vi "Meter Detection Main Page.vi"(8 "error in (no error)":errorcluster, 11 "Node Ptr":T2 format="%.0x") -> (0 "error out":errorcluster)   [LabVIEW 2011, in "Meter Detection Custom Device.lvlib"]
uses:
  Meter Detection Custom Device.lvlib
  <vilib>/NI Veristand/Custom Device API/Custom Device Item Ref.ctl
  <vilib>/NI Veristand/Custom Device API/Custom Device API.lvlib
  <vilib>/vision/driver/NI_Vision_Acquisition_Software.lvlib
panel:
  in  "Needle Configuration":bool
  in  "Reset Max":bool
  in  "Max Meter Value":dbl
  in  "Set Max Meter ROI":bool
  out "Instructions for Use":string
  in  "Reset Min":bool
  in  "Min Meter Value":dbl
  in  "Camera Interface":string
  in  "Set Min Meter ROI":bool
  in  "Capture Image":bool
  out "Image":T1(plugin-control)
  in  "Header":cluster{"Section Name":string}={"Section Name"="Custom Device Item Settings"}
  in  "Name":string
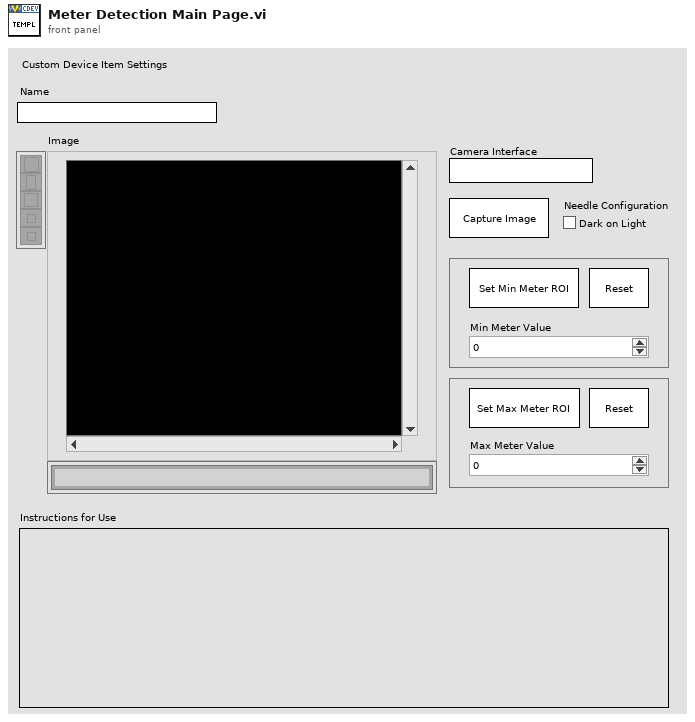
[diagram p1: front panel]
types:
  T1 = typedef "IMAQ Image.ctl" = refnum<image>
  T2 = typedef "Custom Device API.lvlib/Custom Device Item Ref.ctl" = u64
  T3 = typedef "Custom Device API.lvlib/Custom Device Item Info.ctl" = cluster{"Name":string, "Is Channel":bool, "GUID":string}
  T4 = typedef "IMAQdx.ctl" = refnum<k21>
  T5 = cluster{"Global Rectangle":i32[], "Contours":cluster{"Contour Type":u32, "ROI Type":u32, "Points":i32[]}[]}
  T6 = typedef "Custom Device API.lvlib/Custom Device Commands.ctl" = enum16{"Default", "Item renamed", "Shutdown", "Dynamic button pressed"}
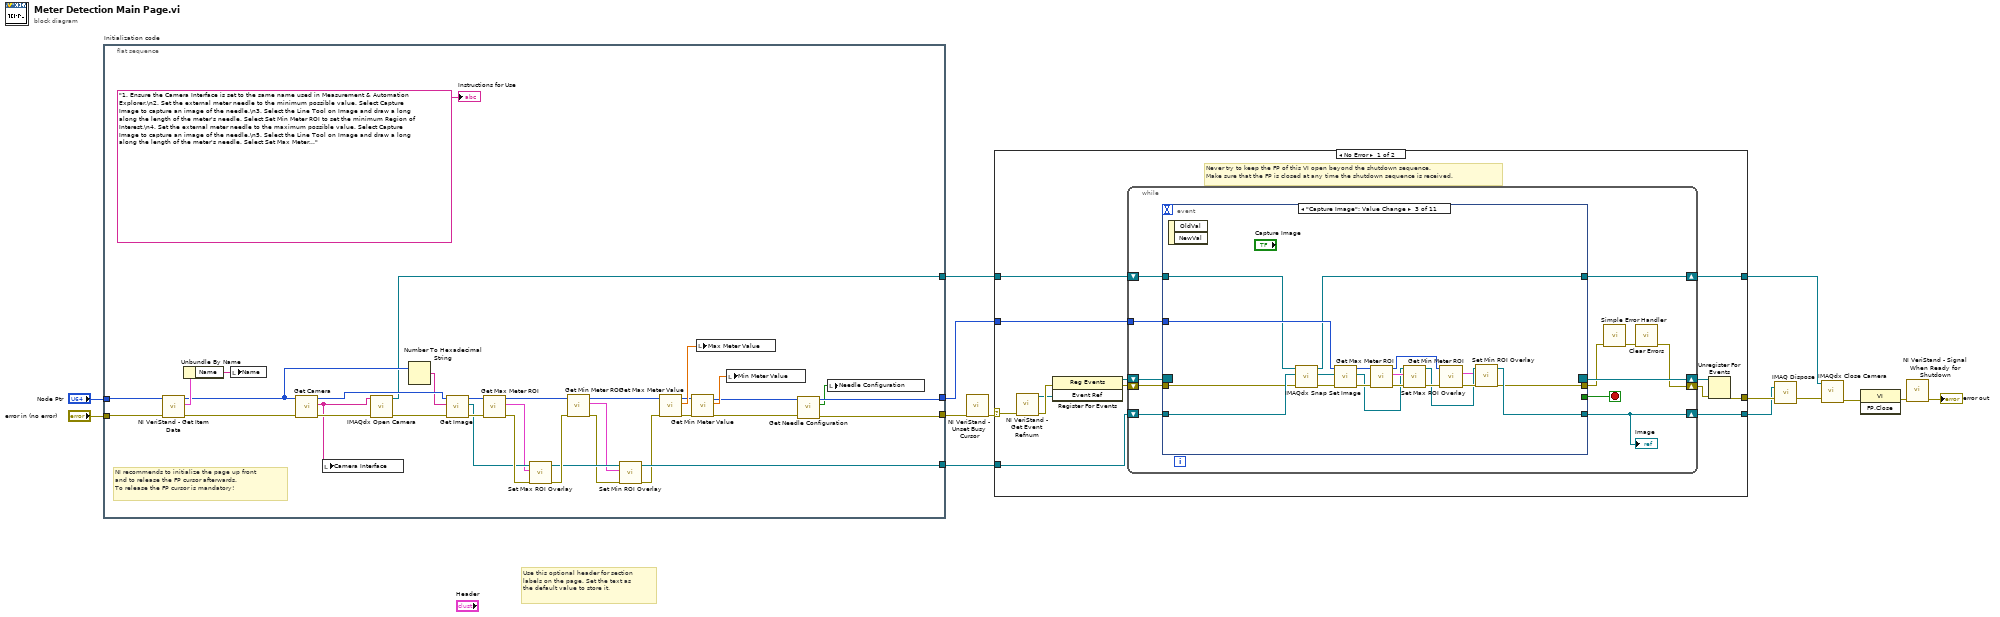
[diagram p0: block diagram]
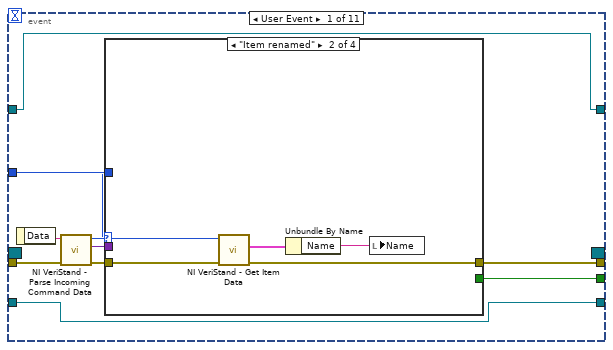
[diagram p2: hidden frame]
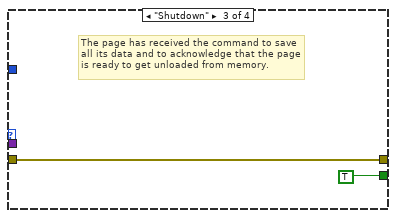
[diagram p4: hidden frame]
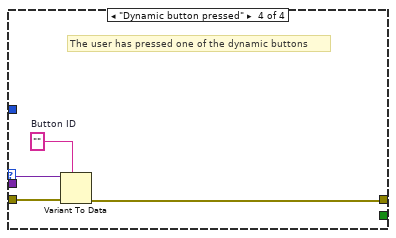
[diagram p5: hidden frame]
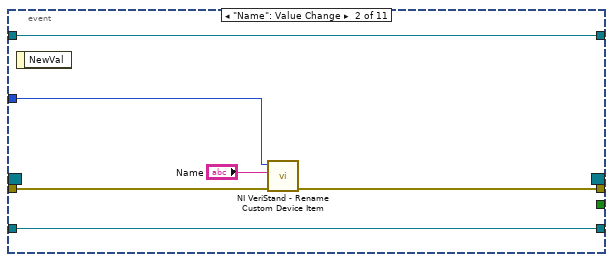
[diagram p6: hidden frame]
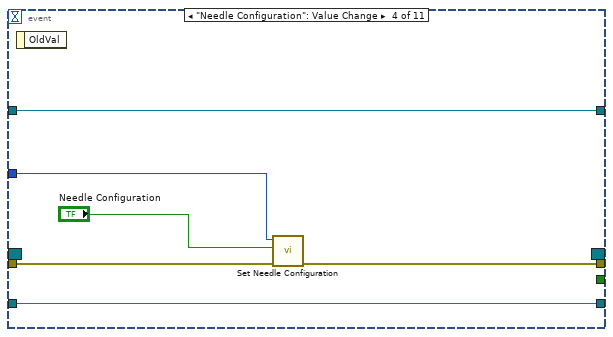
[diagram p7: hidden frame]
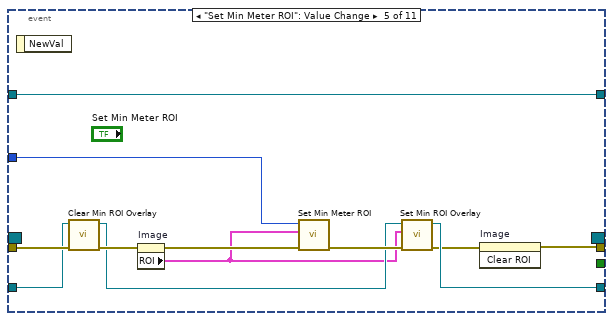
[diagram p8: hidden frame]
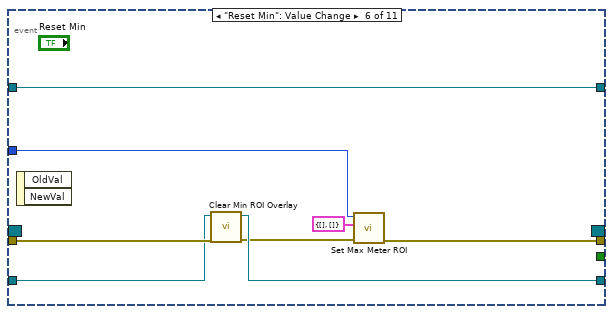
[diagram p9: hidden frame]
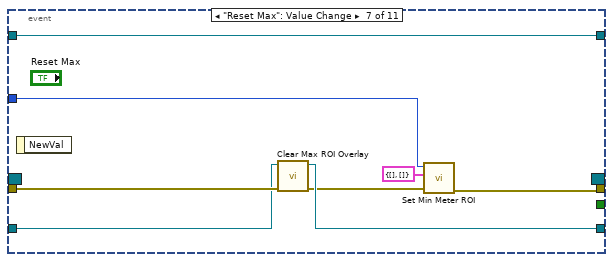
[diagram p10: hidden frame]
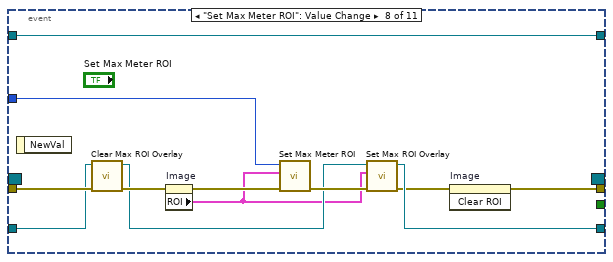
[diagram p11: hidden frame]
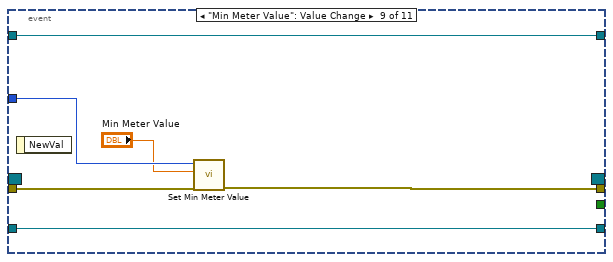
[diagram p12: hidden frame]
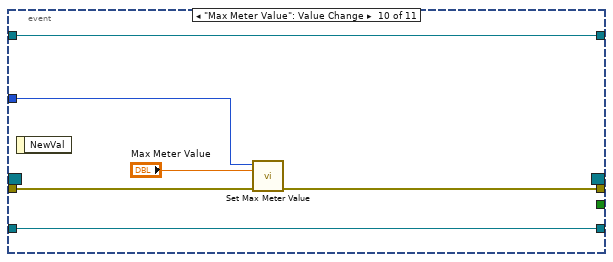
[diagram p13: hidden frame]
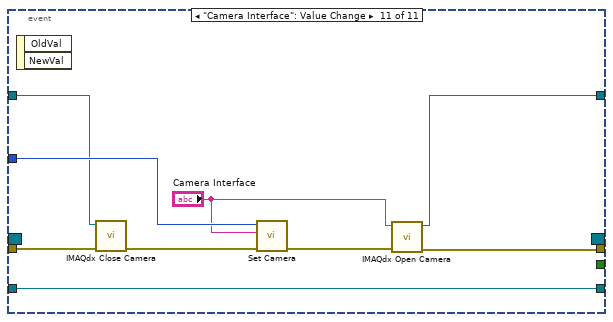
[diagram p14: hidden frame]
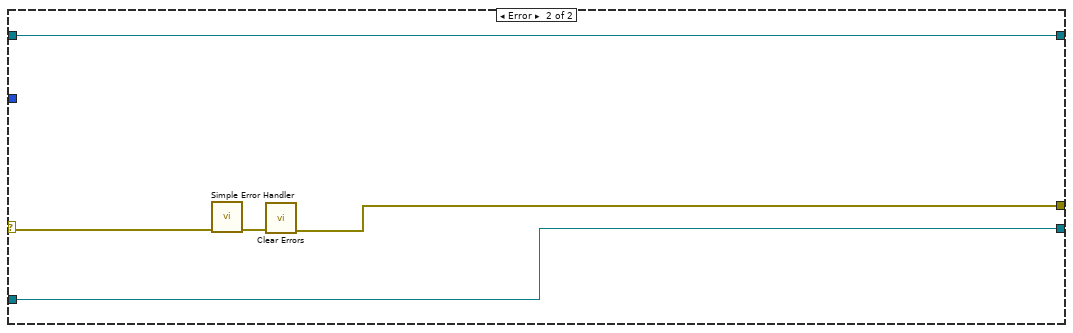
[diagram p15: hidden frame]
diagram:
  # "Use this optional header for section labels on the page. Set the text as the default value to store it."
  n1 = flat-sequence "Initialization code" {
    tunnel: "error in (no error)" -> [w46]
    tunnel: "Node Ptr" -> [w47]
    tunnel: [w16] -> w11
    tunnel: [w17] -> w8
    tunnel: [w27] -> w5
    tunnel: [w21] -> w4
    frame #0 {
      # "NI recommends to initialize the page up front\nand to release the FP cursor afterwards.\nTo release the FP cursor is mandatory!"
      n2 = call <vilib>:"NI VeriStand - Get Item Data.vi"("error in (no error)"=w46, "Item Ref in"=w47) -> ("error out"=w45:errorcluster, "Item Info"=w49:T3, "Item Ref out"=w41:T2)  [unwired: 7 out]
      n3 = Unbundle By Name(w49) -> ("Name"=w48:string)
      n4 = local write "Name"(w48) -> ()
      n5 = call "Get Camera.vi"("error in (no error)"=w45, "Item Ref out in"=w41) -> ("error out"=w24:errorcluster, "Camera"=w22:string, "Item Ref out out"=w44:T2)  [unwired: 7 in]
      n6 = local write "Camera Interface"(w22) -> ()
      n7 = call <vilib>:"IMAQdx Open Camera.vi"("error in"=w24, "Session In"=w22) -> ("error out"=w23:errorcluster, "Session Out"=w21:T4)  [unwired: 8 in]
      n8 = Number To Hexadecimal String(2:w41) -> (0:w35:string)  [unwired: 1 in]
      n9 = call "Get Image.vi"("error in (no error)"=w23, "Image Name"=w35, "Item Ref out out"=w44) -> ("error out"=w34:errorcluster, "Image out"=w31:T1, "Item Ref out"=w43:T2)  [unwired: 5 in, 1 out]
      n10 = call "Get Max Meter ROI.vi"("error in (no error)"=w34, "Item Ref in"=w43) -> ("error out"=w33:errorcluster, "Max Gauge ROI"=w30:T5, "Item Ref out"=w40:T2)  [unwired: 6 in, 1 out]
      n11 = call "Set Max ROI Overlay.vi"("error in (no error)"=w33, "Max Gauge ROI"=w30, "Image in"=w31) -> ("error out"=w32:errorcluster, "Image out"=w29:T1)  [unwired: 7 in]
      n12 = call "Get Min Meter ROI.vi"("error in (no error)"=w32, "Item Ref in"=w40) -> ("error out"=w28:errorcluster, "Max Gauge ROI"=w25:T5, "Item Ref out"=w39:T2)  [unwired: 6 in, 1 out]
      n13 = call "Set Min ROI Overlay.vi"("error in (no error)"=w28, "Min Gauge ROI"=w25, "Image in"=w29) -> ("error out"=w26:errorcluster, "Image out"=w27:T1)  [unwired: 7 in]
      n14 = call "Get Max Meter Value.vi"("error in (no error)"=w26, "Item Ref in"=w39) -> ("error out"=w38:errorcluster, "Max Gauge Value"=w42:dbl, "Item Ref out"=w37:T2)  [unwired: 7 in]
      n15 = call "Get Min Meter Value.vi"("error in (no error)"=w38, "Item Ref in"=w37) -> ("error out"=w19:errorcluster, "Min Gauge Value"=w36:dbl, "Item Ref out"=w18:T2)  [unwired: 7 in]
      n16 = local write "Max Meter Value"(w42) -> ()
      n17 = local write "Min Meter Value"(w36) -> ()
      n18 = call "Get Needle Configuration.vi"("error in (no error)"=w19, "Item Ref in"=w18) -> ("error out"=w16:errorcluster, "Needle Configuration out"=w15:bool, "Item Ref out"=w17:T2)  [unwired: 7 in]
      n19 = local write "Needle Configuration"(w15) -> ()
      "Instructions for Use" <- "1. Ensure the Camera Interface is set to the same name used in Measurement & Automation Explorer.\n2. Set the external meter needle to the minimum possible value. Select Capture Image to capture an image of the needle.\n3. Select the Line Tool on Image and draw a long along the length of the meter's needle. Select Set Min Meter ROI to set the minimum Region of Interest.\n4. Set the external meter needle to the maximum possible value. Select Capture Image to capture an image of the needle.\n5. Select the Line Tool on Image and draw a long along the length of the meter's needle. Select Set Max Meter ROI to set the maximum Region of Interest.\n6. Ensure the Min Meter Value and Max Meter Value correspond to the minimum and maximum possible meter values respectively and set the Needle Configuration appropriately.\n7. Save the system definition file. " ("Directions")
    }
  }
  n20 = call <vilib>:"NI VeriStand - Unset Busy Cursor.vi"("error in (no error)"=w11) -> ("error out"=w10:errorcluster)  [unwired: 10 out]
  n21 = case shown="No Error" w10 {
    selector: w10 -> [w54 w193]
    tunnel: [w59 w191] -> w7
    tunnel: w8 -> [w55 _]
    tunnel: [w53 w190] -> w6
    tunnel: w5 -> [w52 w190]
    tunnel: w4 -> [w51 w189]
    tunnel: [w50 w189] -> w1
    frame No Error {
      # "Never try to keep the FP of this VI open beyond the shutdown sequence.\nMake sure that the FP is closed at any time the shutdown sequence is received."
      n22 = call <vilib>:"NI VeriStand - Get Event Refnum.vi"("error in (no error)"=w54) -> ("error out"=w62:errorcluster, "Event Ref"=w58:refnum<user-event>)  [unwired: 9 out]
      n23 = register-events(error in=w62, w58) -> (reference out=w56:refnum<event-registration>, error out=w57:errorcluster)  [unwired: 1 in]
      n24 = while {
        tunnel: w55 -> [w70]
        shift-right: [w67] -> w60
        shift-left: w57 -> [w73]
        shift-right: [w74] -> w61
        shift-left: w56 -> [w72]
        shift-right: [w65] -> w53
        shift-left: w52 -> [w66]
        shift-right: [w63] -> w50
        shift-left: w51 -> [w64]
        stop <- w71 stop-if-true
        n25 = event shown="[2] \"Capture Image\": Value Change" {
          selector: w72 -> [_ _ _ _ _ _ _ _ _ _ _]
          dyn-events: [_ _ _ _ _ _ _ _ _ _ _] -> w74
          timeout: _ -> [_ _ _ _ _ _ _ _ _ _ _]
          tunnel: w73 -> [w84 w102 w105 w124 w137 w147 w155 w165 w170 w178 w186]
          tunnel: [w80 _ _ _ _ _ _ _ _ _ _] -> w71
          tunnel: [w79 w101 w104 w123 w129 w143 w151 w157 w171 w177 w180] -> w69
          tunnel: w70 -> [w78 w100 w119 w125 w138 w142 w150 w166 w172 w175 w188]
          tunnel: w66 -> [w76 w98 w121 w122 w135 w146 w154 w163 w173 w179 w187]
          tunnel: [w76 w98 w107 w122 w132 w145 w153 w160 w173 w179 w187] -> w65
          tunnel: w64 -> [w75 w97 w106 w127 w128 w140 w148 w156 w168 w174 w184]
          tunnel: [w75 w97 w103 w127 w128 w140 w148 w156 w168 w174 w181] -> w63
          event User Event {
            n26 = event-data() -> ("Data"=w83:string)  [unwired: 1 out]
            n27 = call <vilib>:"NI VeriStand - Parse Incoming Command Data.vi"("error in (no error)"=w84, "Incoming data"=w83) -> ("error out"=w82:errorcluster, "Outgoing data"=w77:variant, "Action"=w81:T6)  [unwired: 7 out]
            n28 = case shown="\"Item renamed\"" w81 {
              tunnel: w82 -> [w85 w90 w91 w96]
              tunnel: [_ _ TRUE _] -> w80
              tunnel: [w85 w87 w91 w93] -> w79
              tunnel: w78 -> [_ w89 _ _]
              tunnel: w77 -> [_ _ _ w95]
              frame "Default", Default {
              }
              frame "Item renamed" {
                n29 = call <vilib>:"NI VeriStand - Get Item Data.vi"("error in (no error)"=w90, "Item Ref in"=w89) -> ("error out"=w87:errorcluster, "Item Info"=w88:T3)  [unwired: 8 out]
                n30 = Unbundle By Name(w88) -> ("Name"=w86:string)
                n31 = local write "Name"(w86) -> ()
              }
              frame "Shutdown" {
                # "The page has received the command to save all its data and to acknowledge that the page is ready to get unloaded from memory."
              }
              frame "Dynamic button pressed" {
                w94 = ""  # Button ID
                # "The user has pressed one of the dynamic buttons"
                n32 = Variant To Data(error in=w96, type=w94, Variant=w95) -> (error out=w93:errorcluster)  [unwired: 1 out]
              }
            }
          }
          event "Name": Value Change {
            n33 = event-data() -> ()  [unwired: 2 out]
            n34 = call <vilib>:"NI VeriStand - Rename Custom Device Item.vi"("error in (no error)"=w102, "New Name"="Name", "Item Ref in"=w100) -> ("error out"=w101:errorcluster)  [unwired: 8 out]
          }
          event "Capture Image": Value Change {
            n35 = event-data() -> ()  [unwired: 3 out]
            n36 = call <vilib>:"IMAQdx Snap.vi"("error in"=w105, "Image In"=w121, "Session In"=w106) -> ("error out"=w120:errorcluster, "Image Out"=w118:T1, "Session Out"=w103:T4)  [unwired: 6 in]
            n37 = call "Set Image.vi"("error in (no error)"=w120, "Image in"=w118, "Item Ref in"=w119) -> ("error out"=w117:errorcluster, "Image out"=w113:T1, "Item Ref out"=w116:T2)  [unwired: 6 in]
            n38 = call "Get Max Meter ROI.vi"("error in (no error)"=w117, "Item Ref in"=w116) -> ("error out"=w115:errorcluster, "Max Gauge ROI"=w114:T5, "Item Ref out"=w111:T2)  [unwired: 6 in, 1 out]
            n39 = call "Set Max ROI Overlay.vi"("error in (no error)"=w115, "Max Gauge ROI"=w114, "Image in"=w113) -> ("error out"=w112:errorcluster, "Image out"=w109:T1)  [unwired: 7 in]
            n40 = call "Get Min Meter ROI.vi"("error in (no error)"=w112, "Item Ref in"=w111) -> ("error out"=w110:errorcluster, "Max Gauge ROI"=w108:T5)  [unwired: 6 in, 2 out]
            n41 = call "Set Min ROI Overlay.vi"("error in (no error)"=w110, "Min Gauge ROI"=w108, "Image in"=w109) -> ("error out"=w104:errorcluster, "Image out"=w107:T1)  [unwired: 7 in]
          }
          event "Needle Configuration": Value Change {
            n42 = event-data() -> ()  [unwired: 2 out]
            n43 = call "Set Needle Configuration.vi"("error in (no error)"=w124, "Needle Configuration in"="Needle Configuration", "Item Ref in"=w125) -> ("error out"=w123:errorcluster)  [unwired: 6 in, 2 out]
          }
          event "Set Min Meter ROI": Value Change {
            n44 = event-data() -> ()  [unwired: 2 out]
            n45 = call "Clear Min ROI Overlay.vi"("error in (no error)"=w137, "Image in"=w135) -> ("error out"=w136:errorcluster, "Image out"=w133:T1)  [unwired: 8 in]
            n46 = property on="Image" class="ImageControl"(error in=w136) -> (error out=w139:errorcluster, "ROI"=w131:T5)  [unwired: 1 in, 1 out]
            n47 = call "Set Min Meter ROI.vi"("error in (no error)"=w139, "ROI"=w131, "Item Ref in"=w138) -> ("error out"=w134:errorcluster)  [unwired: 7 in, 1 out]
            n48 = call "Set Min ROI Overlay.vi"("error in (no error)"=w134, "Min Gauge ROI"=w131, "Image in"=w133) -> ("error out"=w130:errorcluster, "Image out"=w132:T1)  [unwired: 7 in]
            n49 = invoke on="Image" class="ImageControl" method="Clear ROI"(error in=w130) -> (error out=w129:errorcluster)  [unwired: 2 in, 2 out]
          }
          event "Reset Min": Value Change {
            n50 = event-data() -> ()  [unwired: 3 out]
            n51 = call "Clear Min ROI Overlay.vi"("error in (no error)"=w147, "Image in"=w146) -> ("error out"=w144:errorcluster, "Image out"=w145:T1)  [unwired: 8 in]
            n52 = call "Set Max Meter ROI.vi"("error in (no error)"=w144, "ROI"=T5 {"Global Rectangle"=[], "Contours"=[]}, "Item Ref in"=w142) -> ("error out"=w143:errorcluster)  [unwired: 7 in, 1 out]
          }
          event "Reset Max": Value Change {
            n53 = event-data() -> ()  [unwired: 2 out]
            n54 = call "Clear Max ROI Overlay.vi"("error in (no error)"=w155, "Image in"=w154) -> ("error out"=w152:errorcluster, "Image out"=w153:T1)  [unwired: 8 in]
            n55 = call "Set Min Meter ROI.vi"("error in (no error)"=w152, "ROI"=T5 {"Global Rectangle"=[], "Contours"=[]}, "Item Ref in"=w150) -> ("error out"=w151:errorcluster)  [unwired: 7 in, 1 out]
          }
          event "Set Max Meter ROI": Value Change {
            n56 = event-data() -> ()  [unwired: 2 out]
            n57 = call "Clear Max ROI Overlay.vi"("error in (no error)"=w165, "Image in"=w163) -> ("error out"=w164:errorcluster, "Image out"=w161:T1)  [unwired: 8 in]
            n58 = property on="Image" class="ImageControl"(error in=w164) -> (error out=w167:errorcluster, "ROI"=w159:T5)  [unwired: 1 in, 1 out]
            n59 = call "Set Max Meter ROI.vi"("error in (no error)"=w167, "ROI"=w159, "Item Ref in"=w166) -> ("error out"=w162:errorcluster)  [unwired: 7 in, 1 out]
            n60 = call "Set Max ROI Overlay.vi"("error in (no error)"=w162, "Max Gauge ROI"=w159, "Image in"=w161) -> ("error out"=w158:errorcluster, "Image out"=w160:T1)  [unwired: 7 in]
            n61 = invoke on="Image" class="ImageControl" method="Clear ROI"(error in=w158) -> (error out=w157:errorcluster)  [unwired: 2 in, 2 out]
          }
          event "Min Meter Value": Value Change {
            n62 = event-data() -> ()  [unwired: 2 out]
            n63 = call "Set Min Meter Value.vi"("error in (no error)"=w170, "Min Gauge Value"="Min Meter Value", "Item Ref in"=w172) -> ("error out"=w171:errorcluster)  [unwired: 7 in, 1 out]
          }
          event "Max Meter Value": Value Change {
            n64 = event-data() -> ()  [unwired: 2 out]
            n65 = call "Set Max Meter Value.vi"("error in (no error)"=w178, "Min Gauge Value"="Max Meter Value", "Item Ref in"=w175) -> ("error out"=w177:errorcluster)  [unwired: 7 in, 1 out]
          }
          event "Camera Interface": Value Change {
            n66 = event-data() -> ()  [unwired: 3 out]
            n67 = call <vilib>:"IMAQdx Close Camera.vi"("error in"=w186, "Session In"=w184) -> ("error out"=w185:errorcluster)  [unwired: 9 in]
            n68 = call "Set Camera.vi"("error in (no error)"=w185, "Camera"="Camera Interface", "Item Ref in"=w188) -> ("error out"=w183:errorcluster)  [unwired: 7 in, 1 out]
            n69 = call <vilib>:"IMAQdx Open Camera.vi"("error in"=w183, "Session In"="Camera Interface") -> ("error out"=w180:errorcluster, "Session Out"=w181:T4)  [unwired: 8 in]
          }
        }
        "Image" <- w65
        n70 = call <vilib>:"Simple Error Handler.vi"("error in (no error)"=w69) -> ("error out"=w68:errorcluster)  [unwired: 1 in, 7 out]
        n71 = call <vilib>:"Clear Errors.vi"("error in (no error)"=w68) -> ("error out"=w67:errorcluster)  [unwired: 6 out]
      }
      n72 = Unregister For Events(event registration refnum=w61, error in=w60) -> (error out=w59:errorcluster)
    }
    frame Error {
      n73 = call <vilib>:"Simple Error Handler.vi"("error in (no error)"=w193) -> ("error out"=w192:errorcluster)  [unwired: 1 in, 7 out]
      n74 = call <vilib>:"Clear Errors.vi"("error in (no error)"=w192) -> ("error out"=w191:errorcluster)  [unwired: 6 out]
    }
  }
  n75 = call "IMAQ Dispose"("Image"=w6, "error in (no error)"=w7) -> ("error out"=w3:errorcluster)  [unwired: 4 in]
  n76 = call <vilib>:"IMAQdx Close Camera.vi"("error in"=w3, "Session In"=w1) -> ("error out"=w2:errorcluster)  [unwired: 9 in]
  n77 = invoke class="VI" method="FP.Close"(error in=w2) -> (error out=w14:errorcluster)  [unwired: 2 in, 2 out]
  n78 = call <vilib>:"NI VeriStand - Signal When Ready for Shutdown.vi"("error in (no error)"=w14) -> ("error out"=→"error out":errorcluster)  [unwired: 10 out]
